vi "Disable_Relays.vi"(8 "error in (no error)":errorcluster caption="entrée d'erreur (pas d'erreur)", 11 "Class Relay_Board 16_Relay_R4D3D16 en entrée":refnum<class "Class Relay_Board 8_Relay_RY408D.lvclass">) -> (0 "error out":errorcluster caption="sortie d'erreur", 3 "Class Relay_Board 16_Relay_R4D3D16 en sortie":refnum<class "Class Relay_Board 8_Relay_RY408D.lvclass">)   [LabVIEW 2020, in "Library Instrument & Equipement.lvlib" / "Library Relay_Board.lvlib" / "Class Relay_Board 8_Relay_RY408D.lvclass"]
uses:
  Class Relay_Board 8_Relay_RY408D.lvclass
  C:/Users/ngarcin/OneDrive - Altyor/Standard TB/Class/Relay_Board/Relay_Board (Default)/Class Relay_Board (Default).lvclass
  Class Relay_Board 8_Relay_RY408D.lvclass/Class Relay_Board 8_Relay_RY408D.ctl
  Commun VI/TypeDef/Liste Error.ctl
  Commun VI/Library Commun.lvlib
  Modbus/Modbus.lvclass
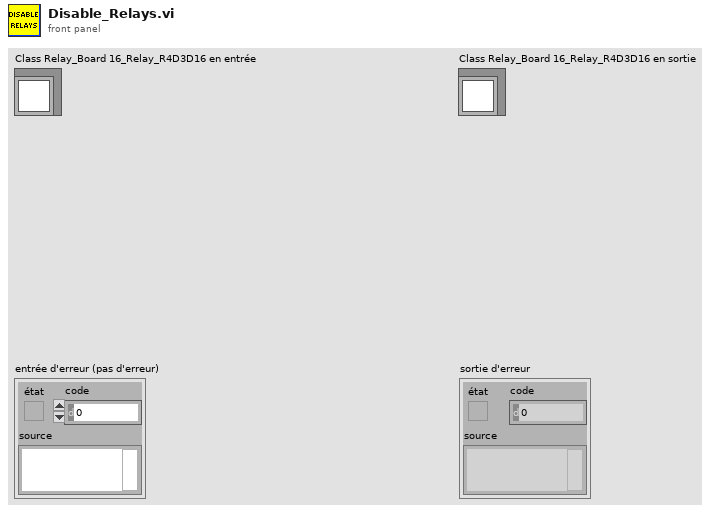
[diagram p1: front panel]
types:
  T1 = typedef "Library Commun.lvlib/Liste Error.ctl" = enum16{"Firebase Driver - Get Document", "Firebase Driver - Get Document With Where", "Firebase Driver - Delete Document", "Firebase Driver - Set Document", "Firebase Driver - Update Document", "Firebase Altyor - Search Document Bench", "Firebase Altyor - Class Not in Firebase", "Spectrum_Analyser - Timeout", "Relay Board - Qty Relay", "DIO - Pb Funtion", "Power_Supply - Peripherical not find", "Mutimeter - Peripherical not find", "Instrument - Function Not Used", "Instrument - Instrument name not specified", "Instrument - Allready Initialised", "Instrument - TimeOut", "Instrument - the instrument must be Initialise before", "Instrument - Frame Not received", "Instrument - Frame Nok", "Test - Initialise the File_for_Save", "Test - Timeout", "Test - Cmd Error", "FGV - Variable ", "BDD FireBase - Define Class", "SN - Class Not Define"}
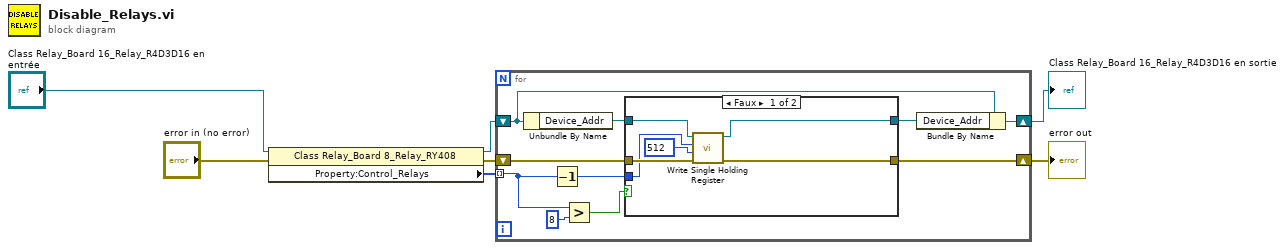
[diagram p0: block diagram]
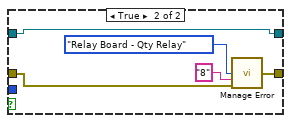
[diagram p2: hidden frame]
diagram:
  n1 = property class="Class Relay_Board 8_Relay_RY408"(reference="Class Relay_Board 16_Relay_R4D3D16 en entrée", error in="error in (no error)") -> (reference out=w2:refnum<class "Class Relay_Board 8_Relay_RY408D.lvclass">, error out=w5:errorcluster, "Property:Control_Relays"=w4:u8[])
  n2 = for {
    shift-right: [w16] -> w7
    shift-left: w5 -> [w17]
    tunnel: w4 -> [w14] mode=indexing
    shift-right: [w10] -> w1
    shift-left: w2 -> [w12]
    n3 = Unbundle By Name(w12) -> ("Device_Addr"=w9:refnum<class "Modbus.lvclass">)
    n4 = Decrement(x=w14) -> (x-1=w8:u8)
    n5 = Greater?(x=w14, y=u8 8) -> (0:w13:bool)
    n6 = case shown="Faux" w13 {
      tunnel: w17 -> [w23 w24]
      tunnel: w8 -> [w22 _]
      tunnel: [w18 w26] -> w16
      tunnel: [w20 w25] -> w11
      tunnel: w9 -> [w19 w25]
      frame False {
        n7 = call "Write Single Holding Register.vi"("error in (no error)"=w23, "value"=u16 512, "address"=w22, "MODBUS in"=w19) -> ("error out"=w18:errorcluster, "MODBUS Out"=w20:refnum<class "Modbus.lvclass">)  [unwired: 6 in]
      }
      frame True {
        n8 = call "Manage Error.vi"("Code Erreur"=Liste_Error."Relay Board - Qty Relay", "Text"="8", "error in (no error)"=w24) -> ("error out"=w26:errorcluster)  [unwired: 12 in]
      }
    }
    n9 = Bundle By Name(cluster=w12, "Device_Addr"=w11) -> (w10:refnum<class "Class Relay_Board 8_Relay_RY408D.lvclass">)
  }
  "error out" <- w7
  "Class Relay_Board 16_Relay_R4D3D16 en sortie" <- w1
